vi "sensor balance2.vi"() -> ()   [LabVIEW 2013]
uses:
  <vilib>/Utility/miscctls.llb/LVBoundsTypeDef.ctl
panel:
  out "연결된 문자열":string
  in  "플롯 영역:크기":T1
  out "XY 그래프 2":cluster{"X":dbl, "Y":dbl}[](graph)
  in  "정지":bool
  in  "a 4":dbl=0.16 format="%#_13g"
  in  "a 3":dbl=0.16 format="%#_13g"
  in  "a 2":dbl=0.16 format="%#_13g"
  in  "a 1":dbl=0.16 format="%#_13g"
  out "웨이브폼 차트":cluster{dbl, dbl, dbl, dbl}(graph)
  in  "숫자형 4":dbl
  in  "숫자형 3":dbl format="%.7f"
  in  "숫자형 2":dbl
  in  "숫자형":dbl format="%.7f"
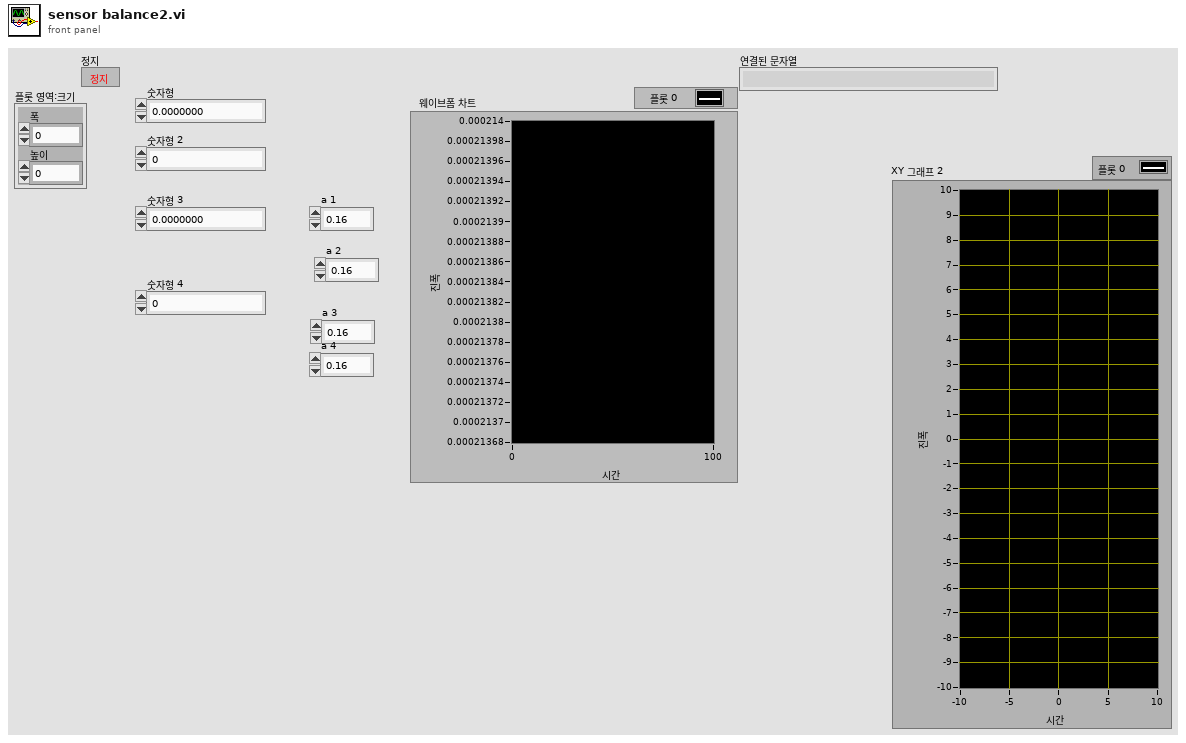
[diagram p1: front panel]
types:
  T1 = typedef "LVBoundsTypeDef.ctl" = cluster{"Width":u32, "Height":u32}
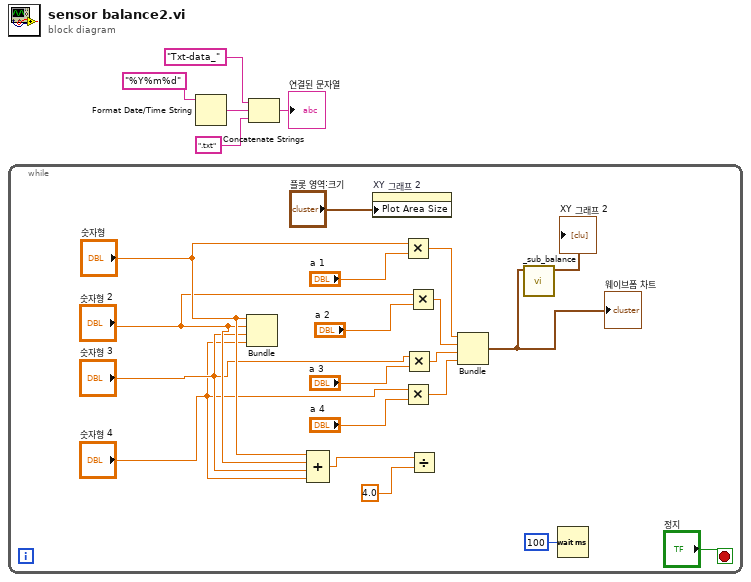
[diagram p0: block diagram]
diagram:
  n1 = while {
    stop <- "정지" stop-if-true
    n2 = Bundle("숫자형"="숫자형", "숫자형 2"="숫자형 2", "숫자형 3"="숫자형 3", "숫자형 4"="숫자형 4") -> ()  [unwired: 1 in, 1 out]
    n3 = Compound Arithmetic op=ADD("숫자형", "숫자형 2", "숫자형 3", "숫자형 4") -> (w9:dbl)
    n4 = property on="XY 그래프 2" class="XYGraph (엄격한)"("Plot Area Size"="플롯 영역:크기") -> ()  [unwired: 2 in, 2 out]
    n5 = Multiply(x="숫자형", y="a 1") -> (x*y=w22:dbl)
    n6 = Multiply(x="숫자형 4", y="a 4") -> (x*y=w16:dbl)
    n7 = Multiply(x="숫자형 3", y="a 3") -> (x*y=w17:dbl)
    n8 = Multiply(x="숫자형 2", y="a 2") -> (x*y=w18:dbl)
    n9 = Divide(x=w9, y=4.0) -> ()  [unwired: 1 out]
    n10 = Bundle(w22, w18, w17, w16) -> (w8:cluster{dbl, dbl, dbl, dbl})  [unwired: 1 in]
    "웨이브폼 차트" <- w8
    n11 = call "_sub_balance.vi"("클러스터"=w8) -> ("Balance"=→"XY 그래프 2":cluster{"X":dbl, "Y":dbl}[])  [unwired: 9 in, 1 out]
    n12 = Wait (ms)(milliseconds to wait=u32 100 ("대기 시간(ms)")) -> ()  [unwired: 1 out]
  }
  n13 = Format Date/Time String(time format string (%c)="%Y%m%d" ("시간 포맷 문자열 (%c)")) -> (date/time string=w3:string)  [unwired: 2 in]
  n14 = Concatenate Strings("Txt-data_" ("이름 또는 상대 경로"), w3, ".txt" ("문자열")) -> (→"연결된 문자열":string)
